vi "SQLProcedureCols.vi"(4 "error in (no error)":errorcluster, 6 "ProcName":string, 7 "InputHandle":i32) -> (0 "error out":errorcluster, 3 "OutputHandle":i32)   [LabVIEW 2011]
doc: "Charge la liste des attributs des requêtes (fonction du catalogue)"
uses:
  Odbc32.dll
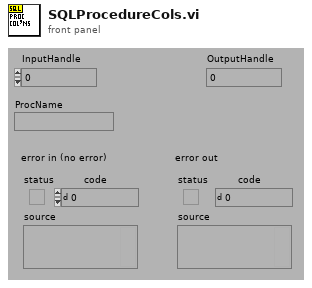
[diagram p1: front panel]
types:
  T1 = enum16{"NOPE", "SQL_HANDLE_ENV", "SQL_HANDLE_DBC", "SQL_HANDLE_STMT", "SQL_HANDLE_DESC"}
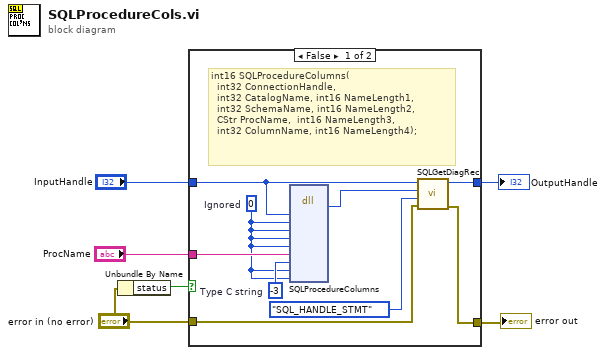
[diagram p0: block diagram]
diagram:
  n1 = Unbundle By Name("error in (no error)") -> ("status"=w1:bool)
  n2 = case shown="False" w1 {
    tunnel: "ProcName" -> [w14 _]
    tunnel: "InputHandle" -> [w11 w17]
    tunnel: [w10 w17] -> w4
    tunnel: [w9 w16] -> w3
    tunnel: "error in (no error)" -> [w8 w16]
    frame False {
      w15 = i16 -3  # Type C string
      w13 = 0  # Ignored
      # "int16 SQLProcedureColumns(\n  int32 ConnectionHandle, \n  int32 CatalogName, int16 NameLength1, \n  int32 SchemaName, int16 NameLength2, \n  CStr ProcName,  int16 NameLength3, \n  int32 ColumnName, int16 NameLength4);"
      n3 = dll-call lib="Odbc32.dll" fn="SQLProcedureColumns"("ConnectionHandle"=w11, "CatalogName"=w13, "NameLength1"=w13, "SchemaName"=w13, "NameLength2"=w13, "ProcName"=w14, "NameLength3"=w15, "ColumnName"=w13, "NameLength4"=w13) -> (w12:i16)  [unwired: 9 in, 5 out]
      n4 = call "SQLGetDiagRec.vi"("error in (no error)"=w8, "HandleType"=T1."SQL_HANDLE_STMT", "Status (SQL_SUCCESS=0)"=w12, "Input Handle"=w11) -> ("error out"=w9:errorcluster, "Output Handle"=w10:i32)  [unwired: 2 out]
    }
    frame True {
    }
  }
  "OutputHandle" <- w4
  "error out" <- w3
